vi "Test RFC5322.vi"(8 "error in":errorcluster) -> (0 "error out":errorcluster)   [LabVIEW 2013]
uses:
  <vilib>/addons/_JKI Toolkits/Caraya/classes/Test/Test.lvclass
  <vilib>/addons/_JKI Toolkits/Caraya/classes/Assert/Assert.lvclass
  <vilib>/addons/_JKI Toolkits/Caraya/classes/Assert/Assert True.vi
  <vilib>/addons/_JKI Toolkits/Caraya/classes/Assert/Assert False.vi
  source/Timestamp Compare Units -- enum.ctl
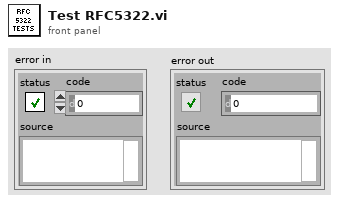
[diagram p1: front panel]
types:
  T1 = typedef "Timestamp Compare Units -- enum.ctl" = enum16{"week", "day", "hour", "minute", "second", "millisecond", "microsecond", "nanosecond"}
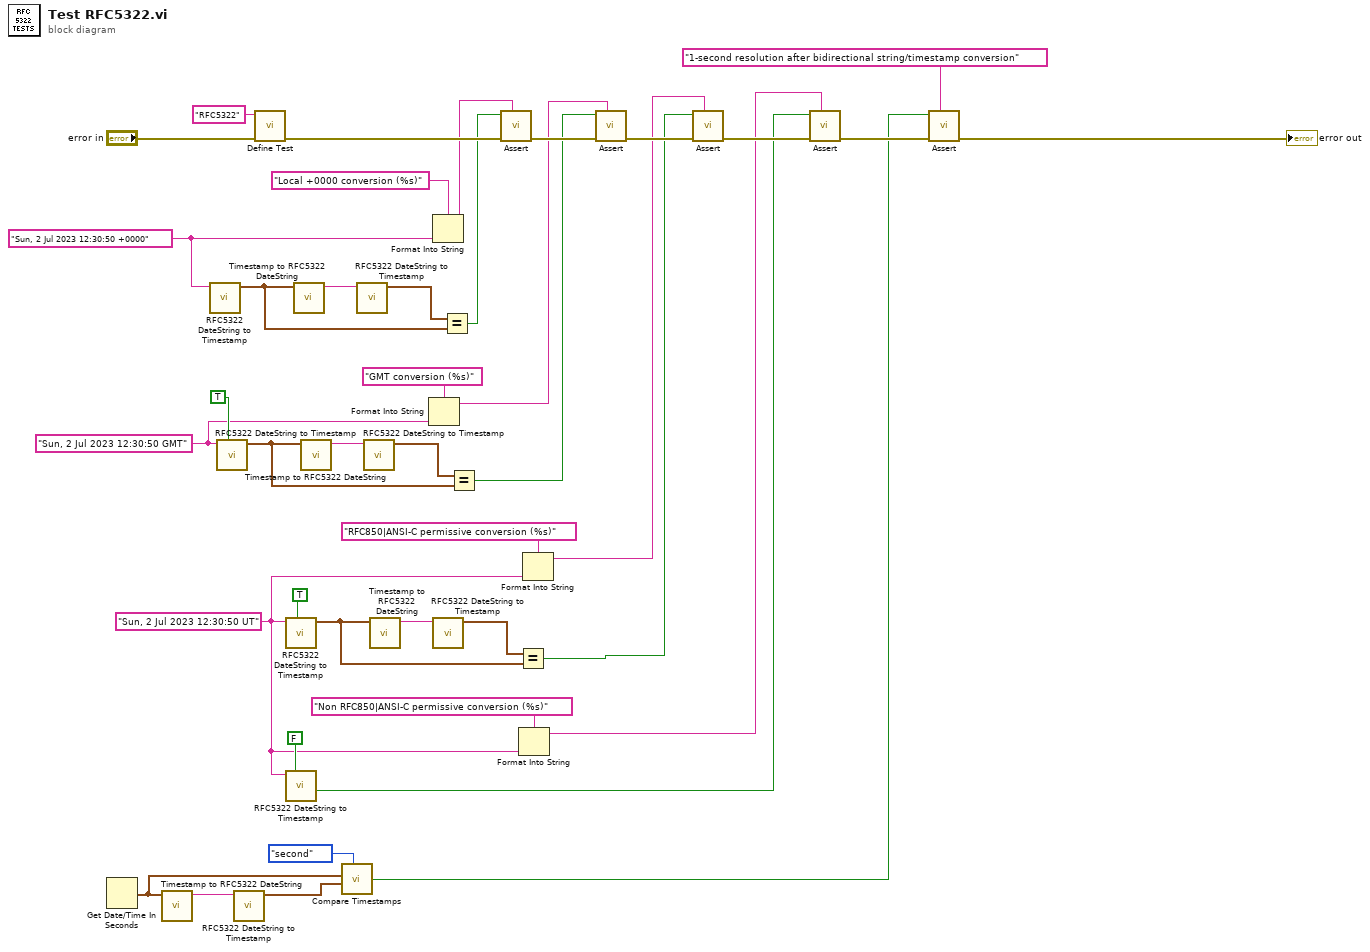
[diagram p0: block diagram]
diagram:
  w12 = "Sun, 2 Jul 2023 12:30:50 UT" ("RFC5322 Date String")
  w19 = "Sun, 2 Jul 2023 12:30:50 GMT" ("RFC5322 Date String")
  w25 = "Sun, 2 Jul 2023 12:30:50 +0000" ("RFC5322 Date String")
  n1 = Get Date/Time In Seconds() -> (seconds since 1Jan1904=w5:timestamp)
  n2 = call "Timestamp to RFC5322 DateString.vi"("Timestamp (now)"=w5) -> ("RFC5322 Date String"=w8:string)  [unwired: 10 in]
  n3 = call "RFC5322 DateString to Timestamp.vi"("RFC5322 String"=w25) -> ("Timestamp"=w36:timestamp)  [unwired: 8 in, 2 out]
  n4 = call "RFC5322 DateString to Timestamp.vi"("RFC850|ANSI-C permissive?"=TRUE, "RFC5322 String"=w19) -> ("Timestamp"=w35:timestamp)  [unwired: 7 in, 2 out]
  n5 = call "RFC5322 DateString to Timestamp.vi"("RFC5322 String"=w8) -> ("Timestamp"=w6:timestamp)  [unwired: 8 in, 2 out]
  n6 = call <vilib>:"Define Test.vi"("error in (no error)"="error in", "Label (VI Title)"="RFC5322") -> ("error out"=w39:errorcluster)  [unwired: 8 in, 1 out]
  n7 = call "RFC5322 DateString to Timestamp.vi"("RFC850|ANSI-C permissive?"=TRUE, "RFC5322 String"=w12) -> ("Timestamp"=w30:timestamp)  [unwired: 7 in, 2 out]
  n8 = call "RFC5322 DateString to Timestamp.vi"("RFC850|ANSI-C permissive?"=FALSE, "RFC5322 String"=w12) -> ("valid?"=w9:bool)  [unwired: 7 in, 2 out]
  n9 = call "Timestamp to RFC5322 DateString.vi"("Timestamp (now)"=w36) -> ("RFC5322 Date String"=w38:string)  [unwired: 10 in]
  n10 = call "Timestamp to RFC5322 DateString.vi"("Timestamp (now)"=w35) -> ("RFC5322 Date String"=w33:string)  [unwired: 10 in]
  n11 = call "Compare Timestamps.vi"("Unit (ms)"=Timestamp_Compare_Units_--_enum."second", "timestamp (1)"=w5, "timestamp (2)"=w6) -> ("Equal?"=w3:bool)  [unwired: 5 in]
  n12 = call "RFC5322 DateString to Timestamp.vi"("RFC5322 String"=w38) -> ("Timestamp"=w37:timestamp)  [unwired: 8 in, 2 out]
  n13 = call "RFC5322 DateString to Timestamp.vi"("RFC5322 String"=w33) -> ("Timestamp"=w34:timestamp)  [unwired: 8 in, 2 out]
  n14 = call "Timestamp to RFC5322 DateString.vi"("Timestamp (now)"=w30) -> ("RFC5322 Date String"=w32:string)  [unwired: 10 in]
  n15 = Format Into String(format string="GMT conversion (%s)" ("x"), w19) -> (resulting string=w18:string)  [unwired: 2 in, 1 out]
  n16 = Format Into String(format string="Local +0000 conversion (%s)" ("x"), w25) -> (resulting string=w24:string)  [unwired: 2 in, 1 out]
  n17 = call "RFC5322 DateString to Timestamp.vi"("RFC5322 String"=w32) -> ("Timestamp"=w31:timestamp)  [unwired: 8 in, 2 out]
  n18 = Equal?(x=w37, y=w36) -> (x = y?=w26:bool)
  n19 = Equal?(x=w34, y=w35) -> (x = y?=w21:bool)
  n20 = call-poly <vilib>:"Assert.vi"("Label"=w24, "error in (no error)"=w39, "True?"=w26) -> ("error out"=w22:errorcluster)  [unwired: 7 in, 1 out]
  n21 = Equal?(x=w31, y=w30) -> (x = y?=w15:bool)
  n22 = Format Into String(format string="Non RFC850|ANSI-C permissive conversion (%s)" ("x"), w12) -> (resulting string=w10:string)  [unwired: 2 in, 1 out]
  n23 = Format Into String(format string="RFC850|ANSI-C permissive conversion (%s)" ("x"), w12) -> (resulting string=w13:string)  [unwired: 2 in, 1 out]
  n24 = call-poly <vilib>:"Assert.vi"("Label"=w18, "error in (no error)"=w22, "True?"=w21) -> ("error out"=w17:errorcluster)  [unwired: 7 in, 1 out]
  n25 = call-poly <vilib>:"Assert.vi"("Label"=w13, "error in (no error)"=w17, "True?"=w15) -> ("error out"=w16:errorcluster)  [unwired: 7 in, 1 out]
  n26 = call-poly <vilib>:"Assert.vi"("Label"=w10, "error in (no error)"=w16, "False?"=w9) -> ("error out"=w4:errorcluster)  [unwired: 7 in, 1 out]
  n27 = call-poly <vilib>:"Assert.vi"("Label"="1-second resolution after bidirectional string/timestamp conversion" ("x"), "error in (no error)"=w4, "True?"=w3) -> ("error out"=→"error out":errorcluster)  [unwired: 7 in, 1 out]
